vi "Zebra_USBPrint_test.vi"() -> ()   [LabVIEW 2017]
uses:
  <vilib>/Utility/NIReport.llb/Append Report Text (str wrap).vi
  <vilib>/Utility/NIReport.llb/NI_report.lvclass
panel:
  in  "standard input":string
  in  "command line":string
  in  "working directory":path=path "F:/"
  in  "report type":T1(ring)
  out "standard error":string
  out "standard output":string
  out "error out 3":errorcluster
  out "error out 2":errorcluster
  in  "print using cmd printer":bool
  in  "print using default printer":bool
  in  "stop":bool
  out "error out":errorcluster
  in  "String":string="^XA^LH10,10^MD20^AD,12^FO120,60^BC^FD11306005MBWD^FS^XZ"
  out "Printing:Default Printer":string
  out "concatenated string":string
  in  "error in (no error)":errorcluster
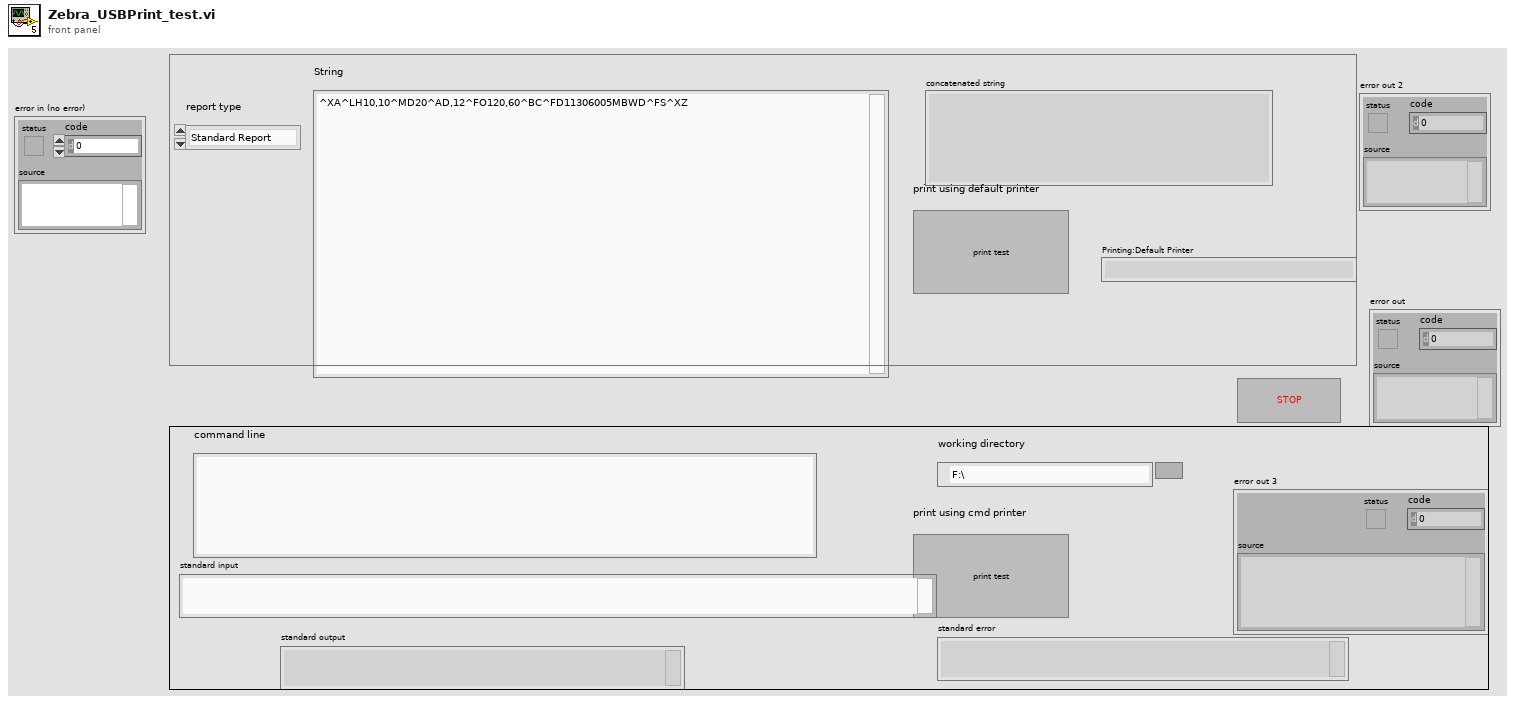
[diagram p1: front panel]
types:
  T1 = enum16{"Standard Report", "HTML", "Word", "Excel"}
  T2 = enum32{"invalid app kind", "Development System", "Run Time System", "Student Edition", "Embedded LabVIEW", "Evaluation", "Custom"}
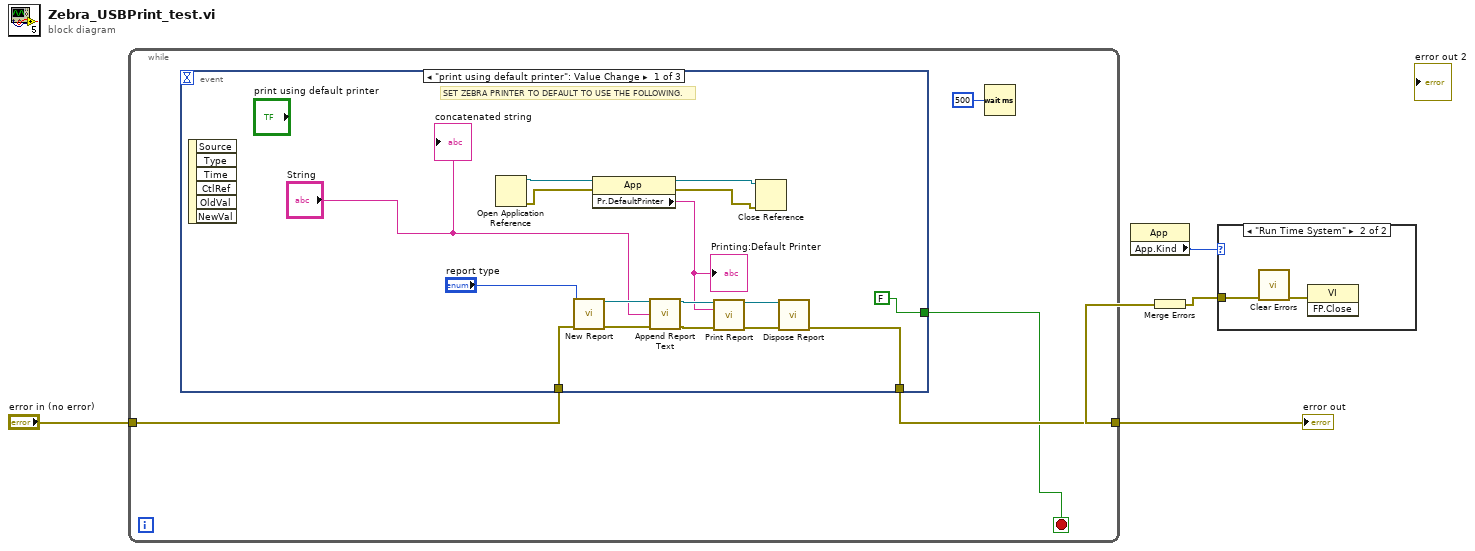
[diagram p0: block diagram]
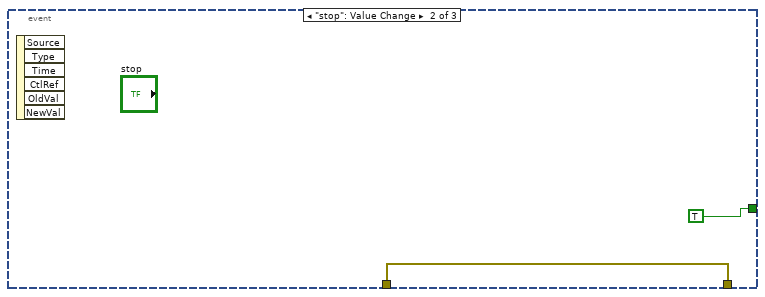
[diagram p3: hidden frame]
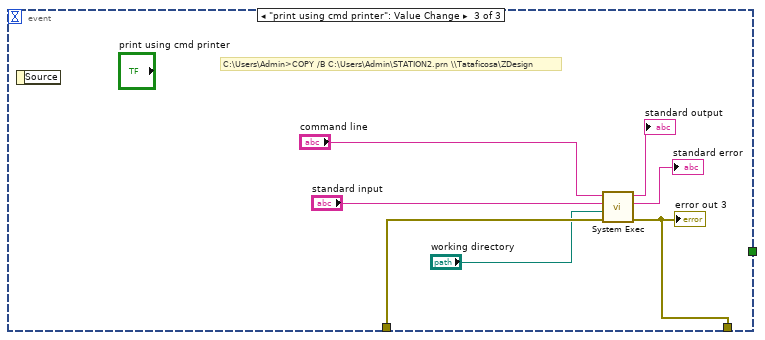
[diagram p4: hidden frame]
diagram:
  n1 = while {
    tunnel: "error in (no error)" -> [w8]
    tunnel: [w7] -> w1
    stop <- w5 stop-if-true
    n2 = event shown="[0] \"print using default printer\": Value Change" {
      selector: _ -> [_ _ _]
      dyn-events: _ -> [_ _ _]
      timeout: _ -> [_ _ _]
      tunnel: w8 -> [w24 w26 w33]
      tunnel: [w11 w26 w32] -> w7
      tunnel: [FALSE TRUE _] -> w5
      event "print using default printer": Value Change {
        # "SET ZEBRA PRINTER TO DEFAULT TO USE THE FOLLOWING."
        n3 = event-data() -> ()  [unwired: 1 in, 6 out]
        n4 = Open Application Reference() -> (0:w20:errorcluster, 3:w23:refnum<vi>)  [unwired: 4 in]
        n5 = call <vilib>:"New Report.vi"("report type"="report type", "error in (no error)"=w24) -> ("report out"=w19:refnum<class "NI_report.lvclass">, "error out"=w18:errorcluster)  [unwired: 12 in]
        n6 = property class="App"(reference=w23, error in=w20) -> (reference out=w22:refnum<vi>, error out=w21:errorcluster, "Pr.DefaultPrinter"=w16:string)
        "Printing:Default Printer" <- w16
        n7 = call-poly <vilib>:"Append Report Text.vi"("report in"=w19, "text"="String", "error in (no error)"=w18) -> ("report out"=w17:refnum<class "NI_report.lvclass">, "error out"=w15:errorcluster)  [unwired: 9 in, 2 out]
        n8 = call-dynamic "Print Report.vi"("report in"=w17, "printer name (default)"=w16, "error in (no error)"=w15) -> ("report out"=w14:refnum<class "NI_report.lvclass">, "error out"=w13:errorcluster)  [unwired: 11 in]
        n9 = Close Reference(reference=w22, error in (no error)=w21) -> ()  [unwired: 1 out]
        n10 = call-dynamic "Dispose Report.vi"("report in"=w14, "error in (no error)"=w13) -> ("error out"=w11:errorcluster)  [unwired: 13 in]
        "concatenated string" <- "String"
      }
      event "stop": Value Change {
        n11 = event-data() -> ()  [unwired: 1 in, 6 out]
      }
      event "print using cmd printer": Value Change {
        # "C:\\Users\\Admin>COPY /B C:\\Users\\Admin\\STATION2.prn \\\\Tataficosa\\ZDesign"
        n12 = event-data() -> ()  [unwired: 1 in, 1 out]
        n13 = call <vilib>:"System Exec.vi"("error in (no error)"=w33, "working directory"="working directory", "standard input"="standard input", "command line"="command line") -> ("error out"=w32:errorcluster, "standard error"=→"standard error":string, "standard output"=→"standard output":string)  [unwired: 4 in, 1 out]
        "error out 3" <- w32
      }
    }
    n14 = Wait (ms)(milliseconds to wait=u32 500) -> ()  [unwired: 1 out]
  }
  "error out" <- w1
  n15 = property class="App"() -> ("App.Kind"=w3:T2)  [unwired: 2 in, 2 out]
  n16 = Merge Errors(w1) -> (w2:errorcluster)
  n17 = case shown="\"Run Time System\"" w3 {
    tunnel: w2 -> [_ w35]
    frame "invalid app kind", Default {
    }
    frame "Run Time System" {
      n18 = call <vilib>:"Clear Errors.vi"("error in (no error)"=w35) -> ("error out"=w34:errorcluster)  [unwired: 5 in, 1 out]
      n19 = invoke class="VI" method="FP.Close"(error in=w34) -> ()  [unwired: 2 in, 3 out]
    }
  }
